vi "svx_Orbit Property Dialog.vi"(6 "Action in":T3 caption="Action", 7 "State in":T4={"X Scale"={"Name"="Horizontal", "FString"="%#.2g", "Major Color"=16777238, "Minor Color"=16777216, "Scale Visible"=TRUE, " Label Visible"=TRUE, "Grid Style"=1}, "Y Scale"={"Name"="Vertical", "FString"="%#.2g", "Major Color"=16777238, "Minor Color"=16777216, "Scale Visible"=TRUE, " Label Visible"=TRUE, "Grid Style"=1}, "Plot"={"Point Style"=0, "Line Width"=0, "Line Style"=0, "Plot Color"=9727, "Point/fill"=0}, "Arrow/Crosshair Color"=9727, "Tacho Point Color"=16711680, "Container Bounds"={"Width"=563, "Height"=294}, "Axis Maximum"=10.0, "Probe Angles"={"Angle X"=0.0, "Angle Y"=1.5707963267948966}, "Background Color"=16777226, "Cursor"={"Cursor Point Style"=13, "Cursor Style"=4, "Cursor Line Width"=1, "Cursor Line Style"=0, "Cursor Color"=9727, "Cursor Name Visible"=TRUE, "Cursor Visible"=TRUE, "Cursor Position"={"X"=0.0, "Y"=0.0}, "Cursor Index"=0, "Cursor Lock"=FALSE}, "Elliptical Info"=[], "Legend Visible"=TRUE, "Scale Range Change"=refnum, "Strings[]"={"Custom pair name"=FALSE, "Row Strings []"=[], "Column Strings []"=[]}, "Index"=[{"pair index"=0, "order index"=0}], " Parents Tags"=[], "Children Tags"=[], "Open?"=[], "Label"="", "Legend Width"=120, "Pair Strings Changed?"=FALSE, "Size"=[], "Legend Background"=16777226, "Legend Font"=16777222, "Cursor Release"=refnum, "Autoscale"=TRUE, "Precession Direction"=[], "Item Width"=0, "User Pair Strings []"=[], "Users Order Strings []"=[], "Autoscale Once"=TRUE, "Property Write"=refnum} caption="State" {"Index"."order index" min=0; "Index"."pair index" min=0; "Axis Maximum" min=0.0}, 8 "Ref In":T1, 11 "Orbit Plot":T2) -> (4 "Action out":T3 caption="Action", 5 "State out":T4={"X Scale"={"Name"="Horizontal", "FString"="%#.2g", "Major Color"=16777238, "Minor Color"=16777216, "Scale Visible"=TRUE, " Label Visible"=TRUE, "Grid Style"=1}, "Y Scale"={"Name"="Vertical", "FString"="%#.2g", "Major Color"=16777238, "Minor Color"=16777216, "Scale Visible"=TRUE, " Label Visible"=TRUE, "Grid Style"=1}, "Plot"={"Point Style"=0, "Line Width"=0, "Line Style"=0, "Plot Color"=9727, "Point/fill"=0}, "Arrow/Crosshair Color"=9727, "Tacho Point Color"=16711680, "Container Bounds"={"Width"=563, "Height"=294}, "Axis Maximum"=10.0, "Probe Angles"={"Angle X"=0.0, "Angle Y"=1.5707963267948966}, "Background Color"=16777226, "Cursor"={"Cursor Point Style"=13, "Cursor Style"=4, "Cursor Line Width"=1, "Cursor Line Style"=0, "Cursor Color"=9727, "Cursor Name Visible"=TRUE, "Cursor Visible"=TRUE, "Cursor Position"={"X"=0.0, "Y"=0.0}, "Cursor Index"=0, "Cursor Lock"=FALSE}, "Elliptical Info"=[], "Legend Visible"=TRUE, "Scale Range Change"=refnum, "Strings[]"={"Custom pair name"=FALSE, "Row Strings []"=[], "Column Strings []"=[]}, "Index"=[{"pair index"=0, "order index"=0}], " Parents Tags"=[], "Children Tags"=[], "Open?"=[], "Label"="", "Legend Width"=120, "Pair Strings Changed?"=FALSE, "Size"=[], "Legend Background"=16777226, "Legend Font"=16777222, "Cursor Release"=refnum, "Autoscale"=TRUE, "Precession Direction"=[], "Item Width"=0, "User Pair Strings []"=[], "Users Order Strings []"=[], "Autoscale Once"=TRUE, "Property Write"=refnum} caption="State" {"Index"."order index" min=0; "Index"."pair index" min=0; "Axis Maximum" min=0.0})   [LabVIEW 2017, in "SVX Orbit.xctl"]
uses:
  <vilib>/addons/_XControls/Orbit Plot/SVX Orbit.xctl
  <vilib>/addons/_XControls/Orbit Plot/subVIs/svx_Orbit Internal State.ctl
  <vilib>/addons/_XControls/Orbit Plot/subVIs/svx_Orbit Bounds.ctl
  <vilib>/_xctls/Action.ctl
  <vilib>/addons/_XControls/Orbit Plot/subVIs/svx_Orbit Data.ctl
  <vilib>/addons/_XControls/Orbit Plot/subVIs/svx_Orbit Core States.ctl
  <vilib>/_xctls/XControlSupport.lvlib
panel:
  in  "Help":bool
  in  "Cancel":bool
  in  "OK":bool
  in  "Main Tab":T6(tab)
  in  "Plot Legend Font.Color":u32(colorbox)=16777222 caption="Legend font"
  in  "Plot Legend Background.Color":u32(colorbox)=16777226 caption="Legend background"
  in  "Background.Color":u32(colorbox) caption="Background"
  in  "Arrow/Crosshair.Color":u32(colorbox)=6618880 caption="Arrow/Crosshair"
  in  "Label.Visible":bool=TRUE
  in  "Label.Text":string="Orbit Plot"
  in  "Caption.Visible":bool
  in  "Caption.Text":string="Orbit Plot"
  in  "Enable State":T7(radio)
  in  "Format Selection":u16(ring) caption="Format selection" items=["Horizontal (X-Axis)", "Vertical (Y-Axis)"]
  in  "Hide trailing zeros":bool=TRUE
  in  "Digits":u8=2
  in  "Precision Type":u16(ring) items=["Digits of precision", "Significant digits"]
  in  "Type":i32(listbox)=2
  in  "Point/Fill.Color":u32(colorbox)=16777226 caption="Point/Fill"
  in  "Plot.Point Style":T8={"OK Button 17"=TRUE, "OK Button"=FALSE, "OK Button 2"=FALSE, "OK Button 3"=FALSE, "OK Button 4"=FALSE, "OK Button 5"=FALSE, "OK Button 6"=FALSE, "OK Button 7"=FALSE, "OK Button 8"=FALSE, "OK Button 9"=FALSE, "OK Button 10"=FALSE, "OK Button 11"=FALSE, "OK Button 12"=FALSE, "OK Button 13"=FALSE, "OK Button 14"=FALSE, "OK Button 15"=FALSE, "OK Button 16"=FALSE} caption="Point Style"
  in  "Line.Color":u32(colorbox) caption="Line"
  in  "Plot.Line Style":T9={"OK Button"=TRUE, "OK Button 2"=FALSE, "OK Button 3"=FALSE, "OK Button 4"=FALSE, "OK Button 5"=FALSE} caption="Line Style"
  in  "Plot.Line Width":T10={"OK Button 2"=TRUE, "OK Button 3"=FALSE, "OK Button 4"=FALSE, "OK Button 5"=FALSE, "OK Button 6"=FALSE, "OK Button 7"=FALSE} caption="Line Width"
  in  "Trigger Point.Color":u32(colorbox)=16711680 caption="Trigger point"
  in  "YGrid Style":u16(ring) caption="Grid Style and Colors"
  in  "XGrid Style":u16(ring) caption="Grid Style and Colors"
  in  "Minor Grid.Color":u32(colorbox)=13056 caption="Minor grid"
  in  "Major Grid.Color":u32(colorbox)=26112 caption="Major grid"
  in  "Scale Label.Visible":bool caption="Show scale label"
  in  "Maximum":dbl=10.0 format="%#.6g"
  in  "Minimum":dbl format="%#.6g"
  in  "Scale Fit":bool caption="Autoscale"
  in  "Scale.Visible":bool=TRUE caption="Show scale"
  in  "Scale Name":string caption="Name"
  in  "Scale Selection":u16(ring) items=["Horizontal (X-Axis)", "Vertical (Y-Axis)"]
  in  "Cursor Info Position.Lock":bool=TRUE
  in  "Cursor.Line Width":T10 caption="Cursor Line Width"
  in  "Cursor.Point Style":T8 caption="Cursor Point Style"
  in  "Cursor.Line Style":T9 caption="Cursor Line Style"
  in  "Cursor Info.Visible":bool caption="Show name"
  in  "Cursor.Style":T11 caption="Cursor Style"
  in  "Cursor.Color":u32(colorbox) caption="Cursor color"
  in  "Cursor.Visible":bool=TRUE
  in  "Tip strip":string
  in  "Description":string
  # "Caption"
  # "Label"
  # "Enabled State"
  # "Color Scheme"
  # "Orbit Plot"
  # "Colors"
  # "Cursor"
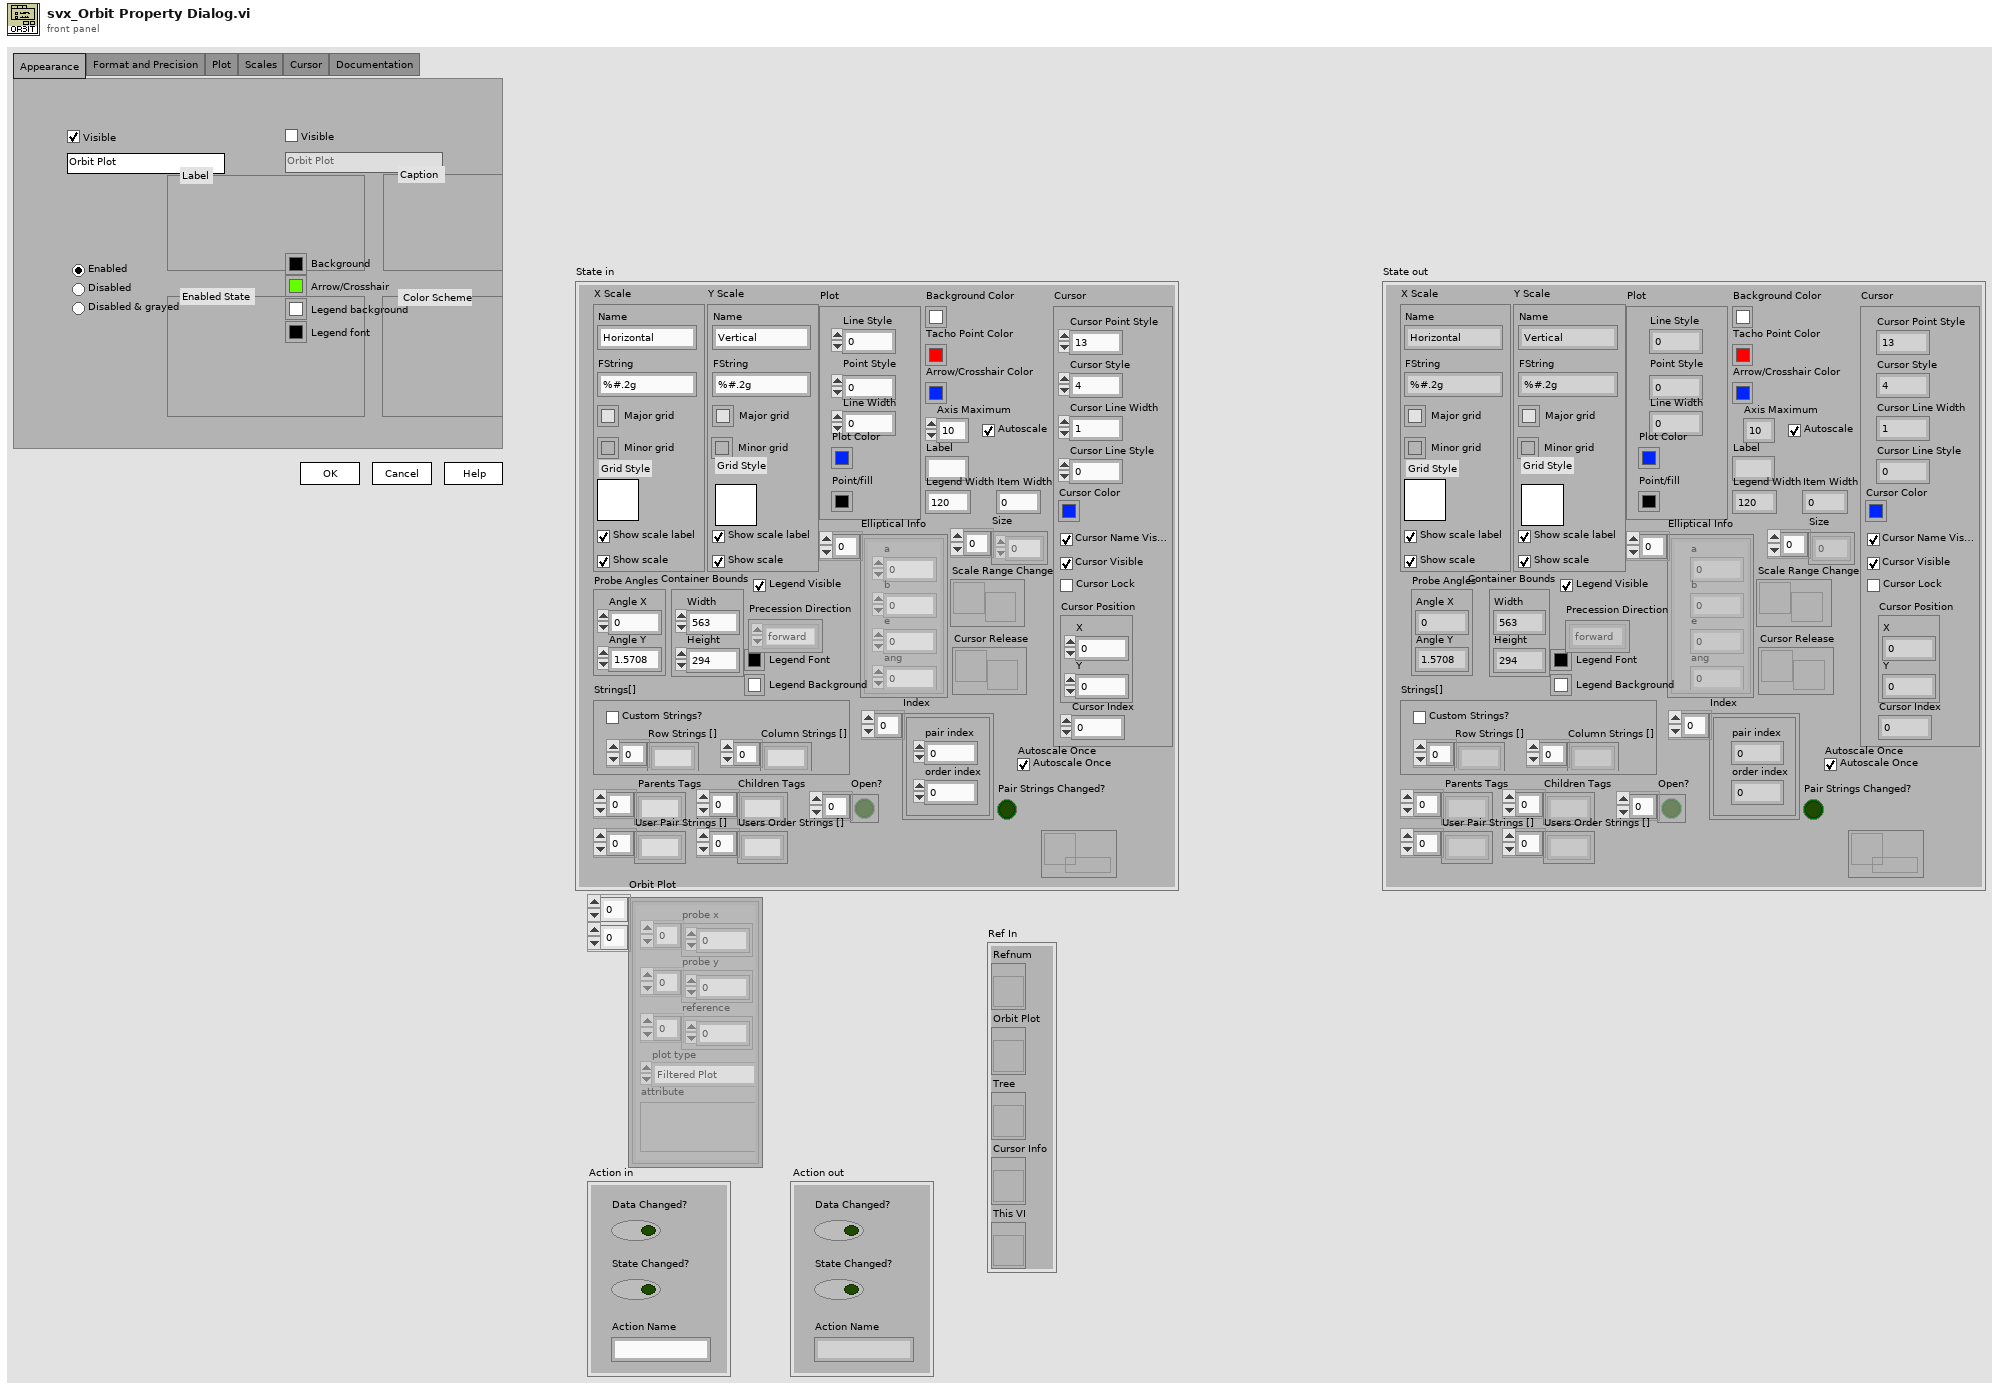
[diagram p1: front panel]
types:
  T1 = cluster{"Refnum":refnum<vi>, "Orbit Plot":refnum<vi>, "Tree":refnum<vi>, "Cursor Info":refnum<vi>, "This VI":refnum<vi>}
  T2 = typedef "SVX Orbit.xctl/svx_Orbit Data.ctl" = cluster{"probe x":dbl[], "probe y":dbl[], "reference":dbl[], "plot type":enum16{"Filtered Plot", "Unfiltered Plot"}, "attribute":variant}[][]
  T3 = typedef "XControlSupport.lvlib/Action.ctl" = cluster{"Data Changed?":bool, "State Changed?":bool, "Action Name":string}
  T4 = typedef "SVX Orbit.xctl/svx_Orbit Internal State.ctl" = cluster{"X Scale":cluster{"Name":string, "FString":string, "Major Color":u32, "Minor Color":u32, "Scale Visible":bool, " Label Visible":bool, "Grid Style":u16}, "Y Scale":cluster{"Name":string, "FString":string, "Major Color":u32, "Minor Color":u32, "Scale Visible":bool, " Label Visible":bool, "Grid Style":u16}, "Plot":cluster{"Point Style":u8, "Line Width":u8, "Line Style":u8, "Plot Color":u32, "Point/fill":u32}, "Arrow/Crosshair Color":u32, "Tacho Point Color":u32, "Container Bounds":T5, "Axis Maximum":dbl, "Probe Angles":cluster{"Angle X":dbl, "Angle Y":dbl}, "Background Color":u32, "Cursor":cluster{"Cursor Point Style":u8, "Cursor Style":u8, "Cursor Line Width":u8, "Cursor Line Style":u8, "Cursor Color":u32, "Cursor Name Visible":bool, "Cursor Visible":bool, "Cursor Position":cluster{"X":dbl, "Y":dbl}, "Cursor Index":i32, "Cursor Lock":bool}, "Elliptical Info":cluster{"a":dbl, "b":dbl, "e":dbl, "ang":dbl}[], "Legend Visible":bool, "Scale Range Change":refnum<user-event>, "Strings[]":cluster{"Custom pair name":bool, "Row Strings []":string[], "Column Strings []":string[]}, "Index":cluster{"pair index":i32, "order index":i32}[], " Parents Tags":string[], "Children Tags":string[], "Open?":bool[], "Label":string, "Legend Width":u32, "Pair Strings Changed?":bool, "Size":i32[], "Legend Background":u32, "Legend Font":u32, "Cursor Release":refnum<user-event>, "Autoscale":bool, "Precession Direction":enum16{"forward", "backward"}[], "Item Width":u32, "User Pair Strings []":string[], "Users Order Strings []":string[], "Autoscale Once":bool, "Property Write":refnum<queue>}
  T5 = typedef "SVX Orbit.xctl/svx_Orbit Bounds.ctl" = cluster{"Width":u32, "Height":u32}
  T6 = enum32{"Appearance", "Format and Precision", "Plot", "Scales", "Cursor", "Documentation"}
  T7 = enum32{"Enabled", "Disabled", "Disabled & grayed"}
  T8 = cluster{"OK Button 17":bool, "OK Button":bool, "OK Button 2":bool, "OK Button 3":bool, "OK Button 4":bool, "OK Button 5":bool, "OK Button 6":bool, "OK Button 7":bool, "OK Button 8":bool, "OK Button 9":bool, "OK Button 10":bool, "OK Button 11":bool, "OK Button 12":bool, "OK Button 13":bool, "OK Button 14":bool, "OK Button 15":bool, "OK Button 16":bool}
  T9 = cluster{"OK Button":bool, "OK Button 2":bool, "OK Button 3":bool, "OK Button 4":bool, "OK Button 5":bool}
  T10 = cluster{"OK Button 2":bool, "OK Button 3":bool, "OK Button 4":bool, "OK Button 5":bool, "OK Button 6":bool, "OK Button 7":bool}
  T11 = cluster{"OK Button 17":bool, "OK Button":bool, "OK Button 2":bool, "OK Button 5":bool, "OK Button 13":bool, "OK Button 10":bool, "OK Button 6":bool, "OK Button 9":bool, "OK Button 14":bool}
  T12 = cluster{"Desc":string, "TipStrip":string, "Label.Text":string, "Label.Visible":bool, "Caption.Text":string, "Caption.Visible":bool, "Disabled":u8}
  T13 = cluster{"probe x":dbl[], "probe y":dbl[], "reference":dbl[], "plot type":enum16{"Filtered Plot", "Unfiltered Plot"}, "attribute":variant}
  T14 = typedef "SVX Orbit.xctl/svx_Orbit Core States.ctl" = enum16{"None", "[Axis] Range", "[Plot] Image", "[Plot] Tacho Point", "[Plot] Grid and BG", "[Cursor] Cursor Info", "[Legend] Pair Strings", "[Data] Plot Data", "[Legend] Checkbox", "[Layout] Update", "[Legend] Tree Open", "[Layout] Legend Visible", "[Plot] Data Point", "[Axis] Axis and Label", "[Axis] Format String", "[Cursor] Appearance", "[Cursor] Index", "[Legend] Color", "[Layout] Min Pane Size", "[Data] Legend Strings"}
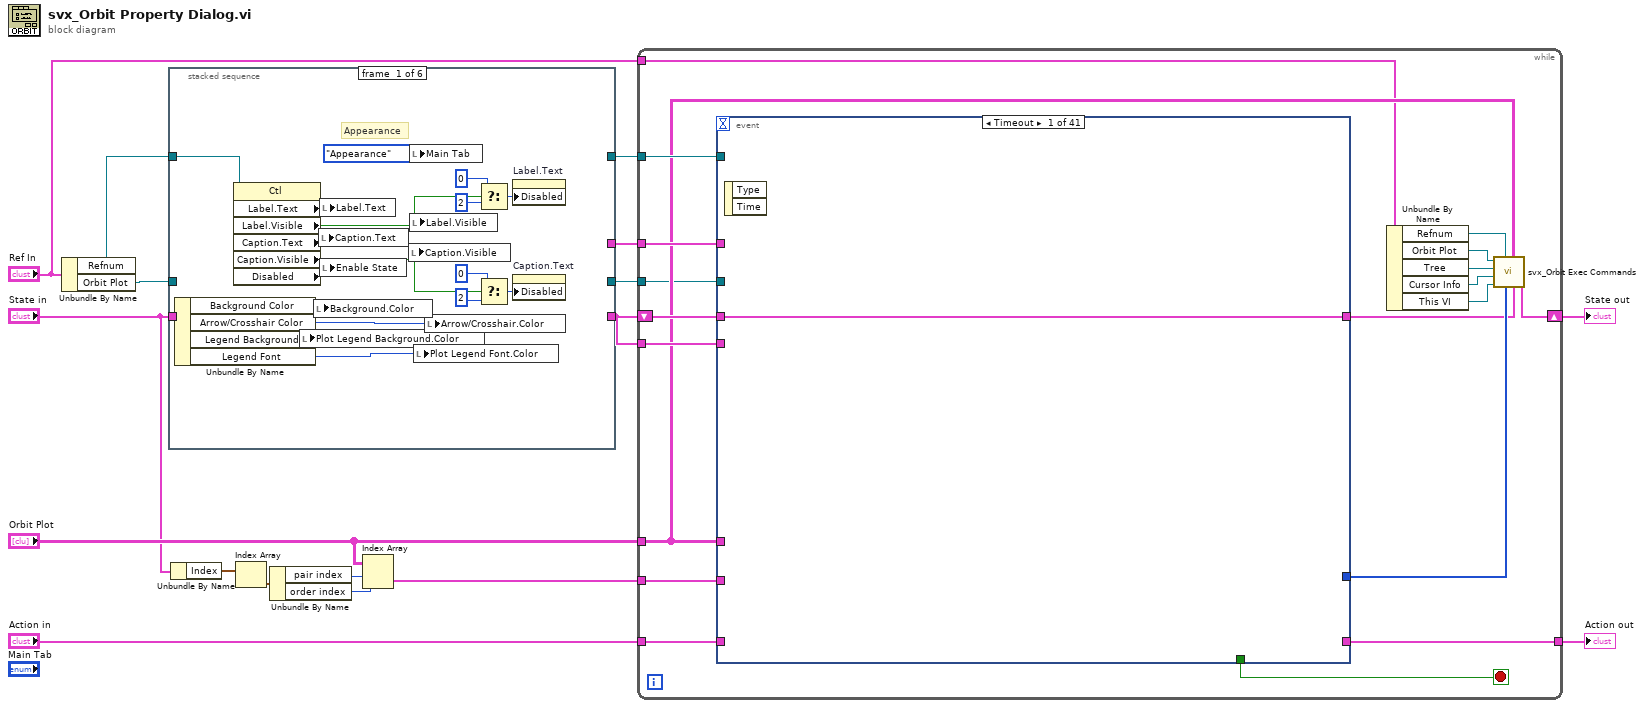
[diagram p0: block diagram]
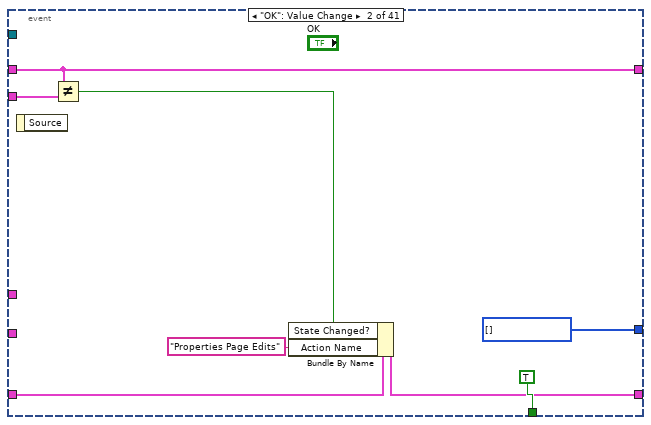
[diagram p2: hidden frame]
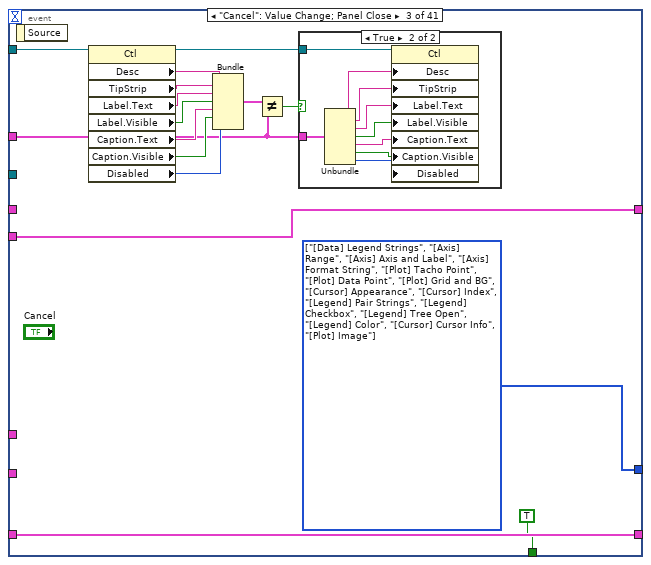
[diagram p3: hidden frame]
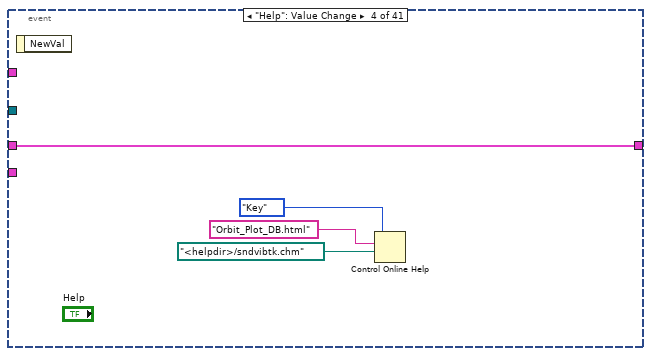
[diagram p5: hidden frame]
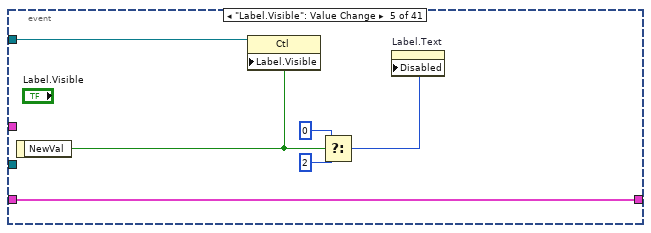
[diagram p6: hidden frame]
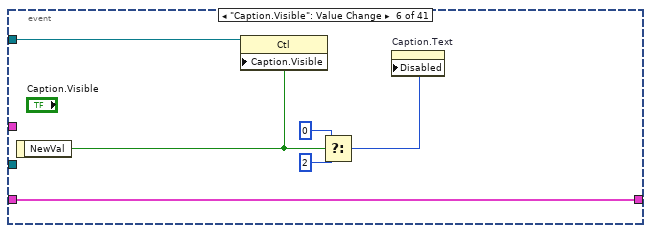
[diagram p7: hidden frame]
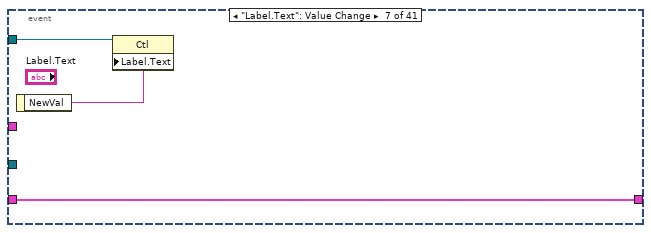
[diagram p8: hidden frame]
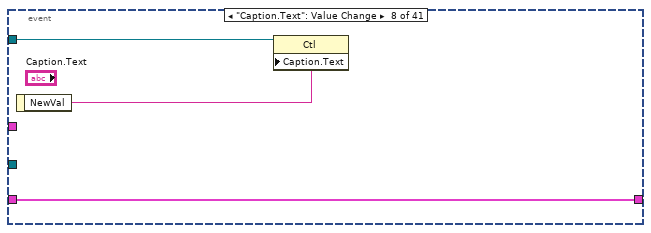
[diagram p9: hidden frame]
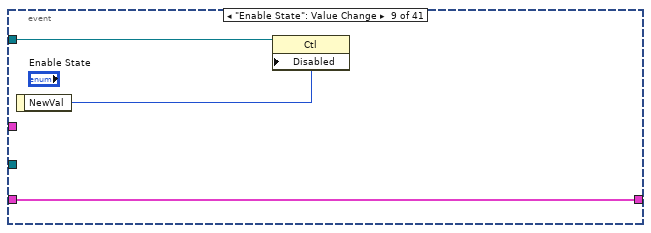
[diagram p10: hidden frame]
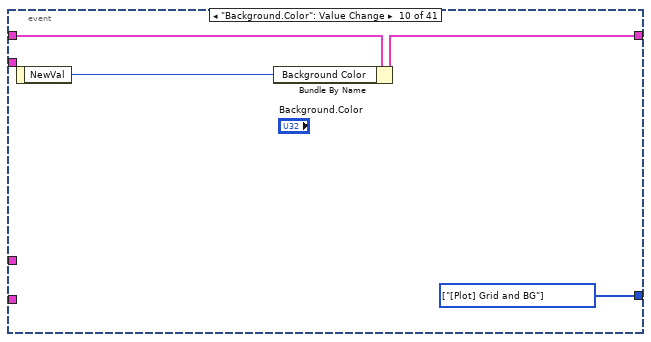
[diagram p11: hidden frame]
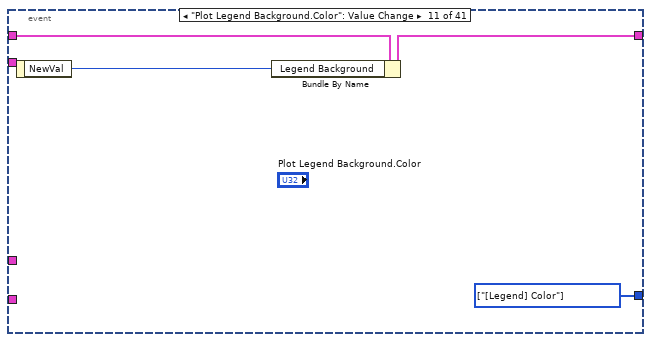
[diagram p12: hidden frame]
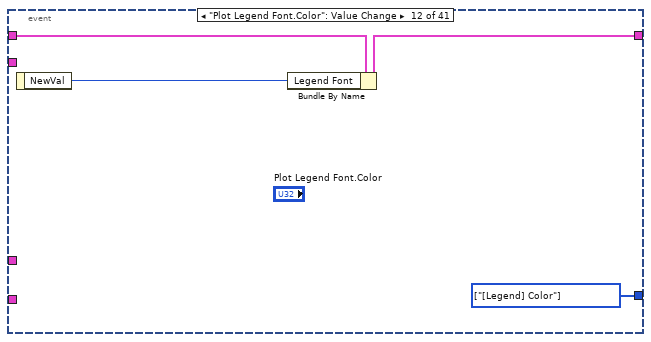
[diagram p13: hidden frame]
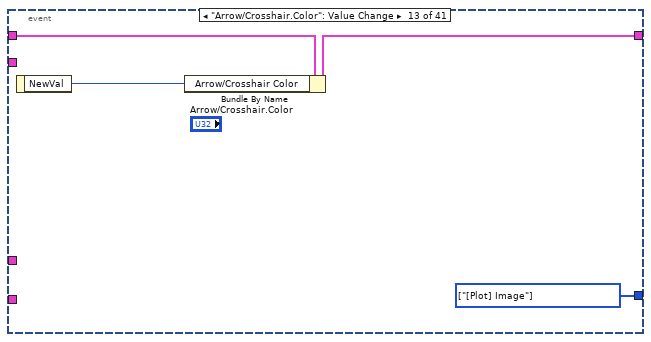
[diagram p14: hidden frame]
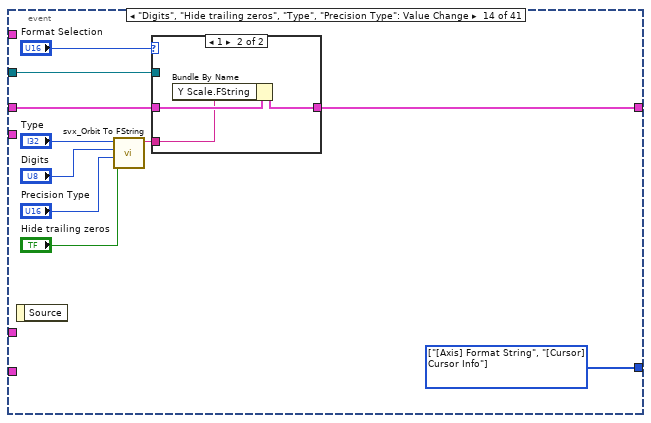
[diagram p15: hidden frame]
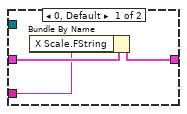
[diagram p16: hidden frame]
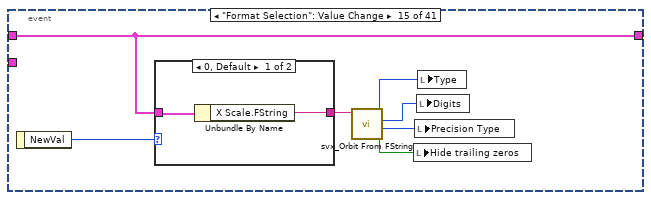
[diagram p17: hidden frame]
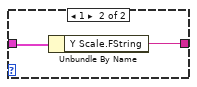
[diagram p18: hidden frame]
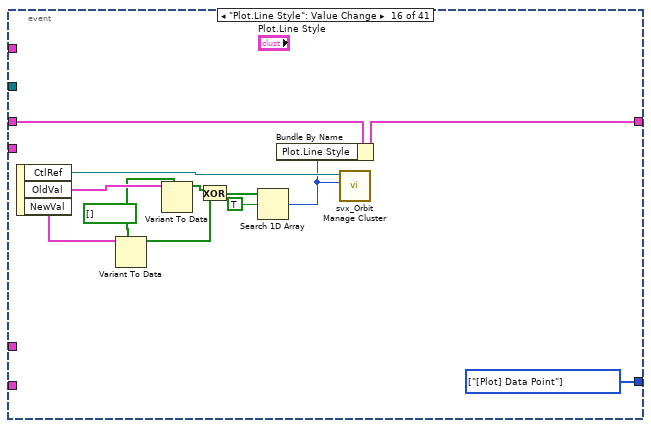
[diagram p19: hidden frame]
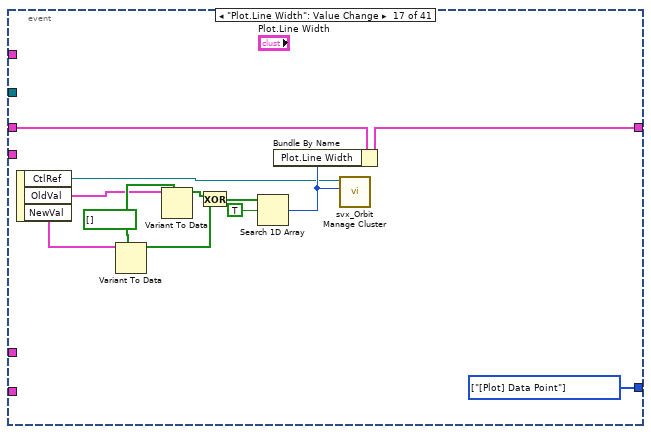
[diagram p20: hidden frame]
diagram:
  n1 = Unbundle By Name("Ref In") -> ("Refnum"=w3:refnum<vi>, "Orbit Plot"=w2:refnum<vi>)
  n2 = stacked-sequence {
    tunnel: w3 -> [w35 _ _ _ _ w118]
    tunnel: "State in" -> [w32 w41 w55 w78 w107 w119]
    tunnel: [_ _ _ _ _ w117] -> w17
    tunnel: [_ _ _ _ _ w119] -> w16
    tunnel: [_ _ _ _ _ w108] -> w14
    tunnel: w2 -> [_ _ _ _ _ w108]
    tunnel: [_ _ _ _ _ w109] -> w13
    frame #0 {
      # "Appearance"
      n3 = Unbundle By Name(w32) -> ("Background Color"=w34:u32, "Arrow/Crosshair Color"=w33:u32, "Legend Background"=w19:u32, "Legend Font"=w18:u32)
      n4 = property class="Ctl"(reference=w35) -> ("Label.Text"=w26:string, "Label.Visible"=w25:bool, "Caption.Text"=w24:string, "Caption.Visible"=w22:bool, "Disabled"=w23:u8)  [unwired: 1 in, 2 out]
      n5 = local write "Plot Legend Background.Color"(w19) -> ()
      n6 = local write "Background.Color"(w34) -> ()
      n7 = local write "Caption.Text"(w24) -> ()
      n8 = local write "Label.Text"(w26) -> ()
      n9 = local write "Enable State"(w23) -> ()
      n10 = local write "Caption.Visible"(w22) -> ()
      n11 = local write "Main Tab"(T6."Appearance" ("Main Tab")) -> ()
      n12 = local write "Label.Visible"(w25) -> ()
      n13 = local write "Plot Legend Font.Color"(w18) -> ()
      n14 = local write "Arrow/Crosshair.Color"(w33) -> ()
      n15 = Select(t=u8 0 ("Disabled"), s=w25, f=u8 2) -> (s? t:f=w30:u8)
      n16 = Select(t=u8 0 ("Disabled"), s=w22, f=u8 2) -> (s? t:f=w27:u8)
      n17 = property on="Label.Text" class="Str"("Disabled"=w30) -> ()  [unwired: 2 in, 2 out]
      n18 = property on="Caption.Text" class="Str"("Disabled"=w27) -> ()  [unwired: 2 in, 2 out]
    }
    frame #1 {
      w42 = u16 0 items=["X-Axis", "Y-Axis"] ("Format selection")
      # "Format and Precision"
      n19 = Unbundle By Name(w41) -> ("X Scale.FString"=w40:string)
      n20 = call <vilib>:"svx_Orbit From FString.vi"("Format string"=w40) -> ("trailing zeros"=w36:bool, "Precision Type"=w37:u16, "Digits"=w38:u8, "Type"=w39:i32)  [unwired: 7 in]
      n21 = local write "Format Selection"(w42) -> ()
      n22 = local write "Hide trailing zeros"(w36) -> ()
      n23 = local write "Precision Type"(w37) -> ()
      n24 = local write "Digits"(w38) -> ()
      n25 = local write "Type"(w39) -> ()
    }
    frame #2 {
      # "Plot"
      n26 = Unbundle By Name(w55) -> ("Plot.Plot Color"=w48:u32, "Tacho Point Color"=w47:u32, "Plot.Point/fill"=w46:u32, "Plot.Line Width"=w54:u8, "Plot.Line Style"=w52:u8, "Plot.Point Style"=w51:u8)
      n27 = control-ref of="Plot.Line Width"() -> (w53:refnum<vi>)
      n28 = control-ref of="Plot.Line Style"() -> (w49:refnum<vi>)
      n29 = control-ref of="Plot.Point Style"() -> (w50:refnum<vi>)
      n30 = To Long Integer(number=w54) -> (32bit integer=w43:i32)
      n31 = To Long Integer(number=w52) -> (32bit integer=w44:i32)
      n32 = To Long Integer(number=w51) -> (32bit integer=w45:i32)
      n33 = local write "Point/Fill.Color"(w46) -> ()
      n34 = local write "Trigger Point.Color"(w47) -> ()
      n35 = call <vilib>:"svx_Orbit Manage Cluster.vi"("index"=w43, "Clust Refnum"=w53) -> ()  [unwired: 10 in]
      n36 = call <vilib>:"svx_Orbit Manage Cluster.vi"("index"=w44, "Clust Refnum"=w49) -> ()  [unwired: 10 in]
      n37 = call <vilib>:"svx_Orbit Manage Cluster.vi"("index"=w45, "Clust Refnum"=w50) -> ()  [unwired: 10 in]
      n38 = local write "Line.Color"(w48) -> ()
    }
    frame #3 {
      w79 = u16 0 items=["X-Axis", "Y-Axis"] ("Scale selection")
      # "Scales"
      n39 = Unbundle By Name(w78) -> ("Y Scale.Name"=w60:string, "X Scale.Name"=w58:string, "X Scale.Label Visible"=w77:bool, "X Scale.Scale Visible"=w76:bool, "X Scale.Grid Style"=w66:u16, "X Scale.Major Color"=w75:u32, "X Scale.Minor Color"=w74:u32, "Autoscale"=w56:bool, "Axis Maximum"=w62:dbl)
      n40 = local write "Scale Selection"(w79) -> ()
      n41 = property on="YGrid Style" class="Ring (strict)"("Visible"=FALSE) -> ()  [unwired: 2 in, 2 out]
      n42 = property on="XGrid Style" class="Ring (strict)"("Visible"=TRUE) -> ()  [unwired: 2 in, 2 out]
      n43 = Concatenate Strings(w60, " (Y-Axis)" ("string")) -> (w63:string)
      n44 = Negate(x=w62) -> (-x=w73:dbl)
      n45 = local write "Minimum"(w73) -> ()
      n46 = local write "Scale Label.Visible"(w77) -> ()
      n47 = local write "Maximum"(w62) -> ()
      n48 = local write "Minor Grid.Color"(w74) -> ()
      n49 = local write "XGrid Style"(w66) -> ()
      n50 = case shown="1" w66 {
        tunnel: [w80 u8 0 ("Disabled") w83] -> w68
        tunnel: [w80 u8 2 ("Disabled") w83] -> w67
        frame 0, Default {
          w80 = u8 2 ("Disabled")
        }
        frame 1 {
        }
        frame 2 {
          w83 = u8 0 ("Disabled")
        }
      }
      n51 = Concatenate Strings(w58, " (X-Axis)" ("string")) -> (w64:string)
      n52 = Build Array(w64, w63) -> (w61:string[])
      n53 = Select(t=u8 2 ("Disabled"), s=w56, f=u8 0) -> (s? t:f=w70:u8)
      n54 = local write "Scale Name"(w58) -> ()
      n55 = local write "Scale.Visible"(w76) -> ()
      n56 = local write "Major Grid.Color"(w75) -> ()
      n57 = local write "Scale Fit"(w56) -> ()
      n58 = property on="Minimum" class="DigNum (strict)"("Disabled"=w70) -> ()  [unwired: 2 in, 2 out]
      n59 = property on="Maximum" class="DigNum (strict)"("Disabled"=w70) -> ()  [unwired: 2 in, 2 out]
      n60 = property on="Major Grid.Color" class="ColBox"("Disabled"=w68) -> ()  [unwired: 2 in, 2 out]
      n61 = property on="Minor Grid.Color" class="ColBox"("Disabled"=w67) -> ()  [unwired: 2 in, 2 out]
      n62 = property on="Format Selection" class="Ring (strict)"("Strings []"=w61) -> ()  [unwired: 2 in, 2 out]
      n63 = property on="Scale Selection" class="Ring (strict)"("Strings []"=w61) -> ()  [unwired: 2 in, 2 out]
    }
    frame #4 {
      # "Cursor"
      n64 = Unbundle By Name(w107) -> ("Cursor.Cursor Point Style"=w106:u8, "Cursor.Cursor Style"=w104:u8, "Cursor.Cursor Line Width"=w102:u8, "Cursor.Cursor Line Style"=w100:u8, "Cursor.Cursor Color"=w98:u32, "Cursor.Cursor Name Visible"=w90:bool, "Cursor.Cursor Visible"=w89:bool, "Cursor.Cursor Lock"=w97:bool)
      n65 = And(x=w90, y=w89) -> (x .and. y?=w88:bool)
      n66 = local write "Cursor Info Position.Lock"(w97) -> ()
      n67 = local write "Cursor Info.Visible"(w90) -> ()
      n68 = To Long Integer(number=w104) -> (32bit integer=w85:i32)
      n69 = To Long Integer(number=w100) -> (32bit integer=w87:i32)
      n70 = control-ref of="Cursor.Point Style"() -> (w105:refnum<vi>)
      n71 = control-ref of="Cursor.Style"() -> (w103:refnum<vi>)
      n72 = control-ref of="Cursor.Line Style"() -> (w99:refnum<vi>)
      n73 = Select(t=u8 0 ("Disabled"), s=w89, f=u8 2) -> (s? t:f=w94:u8)
      n74 = Select(t=u8 0 ("Disabled"), s=w88, f=u8 2) -> (s? t:f=w93:u8)
      n75 = call <vilib>:"svx_Orbit Manage Cluster.vi"("index"=w85, "Clust Refnum"=w103) -> ()  [unwired: 10 in]
      n76 = call <vilib>:"svx_Orbit Manage Cluster.vi"("index"=w87, "Clust Refnum"=w99) -> ()  [unwired: 10 in]
      n77 = To Long Integer(number=w106) -> (32bit integer=w84:i32)
      n78 = To Long Integer(number=w102) -> (32bit integer=w86:i32)
      n79 = control-ref of="Cursor.Line Width"() -> (w101:refnum<vi>)
      n80 = local write "Cursor.Visible"(w89) -> ()
      n81 = local write "Cursor.Color"(w98) -> ()
      n82 = property on="Cursor Info.Visible" class="Bool (strict)"("Disabled"=w94) -> ()  [unwired: 2 in, 2 out]
      n83 = property on="Cursor Info Position.Lock" class="Bool (strict)"("Disabled"=w93) -> ()  [unwired: 2 in, 2 out]
      n84 = call <vilib>:"svx_Orbit Manage Cluster.vi"("index"=w84, "Clust Refnum"=w105) -> ()  [unwired: 10 in]
      n85 = call <vilib>:"svx_Orbit Manage Cluster.vi"("index"=w86, "Clust Refnum"=w101) -> ()  [unwired: 10 in]
    }
    frame #5 {
      n86 = property class="Ctl"(reference=w118) -> (reference out=w117:refnum<vi>, "Desc"=w110:string, "TipStrip"=w111:string, "Label.Text"=w116:string, "Label.Visible"=w115:bool, "Caption.Text"=w114:string, "Caption.Visible"=w113:bool, "Disabled"=w112:u8)  [unwired: 1 in, 1 out]
      n87 = local write "Description"(w110) -> ()
      n88 = local write "Tip strip"(w111) -> ()
      n89 = Bundle("Desc"=w110, "TipStrip"=w111, "Label.Text"=w116, "Label.Visible"=w115, "Caption.Text"=w114, "Caption.Visible"=w113, "Disabled"=w112) -> (w109:T12)  [unwired: 1 in]
    }
  }
  n90 = Unbundle By Name("State in") -> ("Index"=w8:cluster{"pair index":i32, "order index":i32}[])
  n91 = Index Array(array=w8) -> (element=w7:cluster{"pair index":i32, "order index":i32})  [unwired: 1 in]
  n92 = Unbundle By Name(w7) -> ("pair index"=w6:i32, "order index"=w5:i32)
  n93 = Index Array(array="Orbit Plot", index (row)=w6, index (col)=w5) -> (element=w9:T13)
  n94 = while {
    tunnel: w17 -> [w135]
    shift-right: [w129] -> w12
    shift-left: w16 -> [w137]
    tunnel: w16 -> [w133]
    tunnel: w14 -> [w126]
    tunnel: w13 -> [w134]
    tunnel: "Orbit Plot" -> [w128]
    tunnel: w9 -> [w132]
    tunnel: "Action in" -> [w136]
    tunnel: [w127] -> w4
    tunnel: "Ref In" -> [w125]
    stop <- w138 stop-if-true
    n95 = event shown="[0] Timeout" {
      selector: _ -> [_ _ _ _ _ _ _ _ _ _ _ _ _ _ _ _ _ _ _ _ _ _ _ _ _ _ _ _ _ _ _ _ _ _ _ _ _ _ _ _ _]
      dyn-events: _ -> [_ _ _ _ _ _ _ _ _ _ _ _ _ _ _ _ _ _ _ _ _ _ _ _ _ _ _ _ _ _ _ _ _ _ _ _ _ _ _ _ _]
      timeout: _ -> [_ _ _ _ _ _ _ _ _ _ _ _ _ _ _ _ _ _ _ _ _ _ _ _ _ _ _ _ _ _ _ _ _ _ _ _ _ _ _ _ _]
      tunnel: [_ TRUE TRUE _ _ _ _ _ _ _ _ _ _ _ _ _ _ _ _ _ _ _ _ _ _ _ _ _ _ _ _ _ _ _ _ _ _ _ _ _ _] -> w138
      tunnel: w137 -> [w139 w140 _ w173 w177 w183 w189 w192 w195 w201 w205 w209 w212 w216 w235 w244 w259 w271 w280 w284 w288 w297 w310 w321 w331 w343 w349 w359 w369 w380 w389 w435 w447 w459 w471 w483 w485 w499 w503 w504 w507]
      tunnel: w133 -> [_ w146 w161 _ _ _ _ _ _ _ _ _ _ _ _ _ _ _ _ _ _ _ _ _ _ _ _ _ _ _ _ _ _ _ _ _ _ _ _ _ _]
      tunnel: w136 -> [_ w145 w163 _ _ _ _ _ _ _ _ _ _ _ _ _ _ _ _ _ _ _ _ _ _ _ _ _ _ _ _ _ _ _ _ _ _ _ _ _ _]
      tunnel: [_ w144 w163 _ _ _ _ _ _ _ _ _ _ _ _ _ _ _ _ _ _ _ _ _ _ _ _ _ _ _ _ _ _ _ _ _ _ _ _ _ _] -> w127
      tunnel: [_ w141 w160 _ _ _ _ _ _ w198 w202 w206 w210 w214 _ w241 w253 w265 w277 w281 w285 w289 w306 w317 _ w338 w348 w355 w365 w376 _ w429 w441 w453 w465 w477 w486 w496 w500 _ _] -> w131
      tunnel: w126 -> [_ _ _ _ _ _ _ _ _ _ _ _ _ w218 _ _ _ _ _ _ _ _ _ _ w337 _ _ _ _ _ _ _ _ _ _ _ _ _ _ _ _]
      tunnel: w135 -> [_ _ w148 _ w182 w188 w191 w194 w197 _ _ _ _ _ _ _ _ _ _ _ _ _ _ _ _ _ _ _ _ _ _ _ _ _ _ _ _ _ _ w506 w509]
      tunnel: w134 -> [_ _ w149 _ _ _ _ _ _ _ _ _ _ _ _ _ _ _ _ _ _ _ _ _ _ _ _ _ _ _ _ _ _ _ _ _ _ _ _ _ _]
      tunnel: [w139 w140 w161 w173 w177 w183 w189 w192 w195 w200 w203 w208 w213 w215 w235 w243 w258 w270 w279 w283 w287 w296 w309 w320 w329 w340 w350 w360 w368 w379 w389 w434 w446 w458 w470 w482 w495 w498 w501 w504 w507] -> w130
      tunnel: w128 -> [_ _ _ _ _ _ _ _ _ _ _ _ _ _ _ _ _ _ _ _ _ _ _ _ _ _ _ _ _ _ _ _ _ _ _ _ _ _ _ _ _]
      tunnel: w132 -> [_ _ _ _ _ _ _ _ _ _ _ _ _ _ _ _ _ _ _ _ _ _ _ _ w333 _ _ _ _ _ _ _ _ _ _ _ _ _ _ _ _]
      event Timeout {
        n96 = event-data() -> ()  [unwired: 1 in, 2 out]
      }
      event "OK": Value Change {
        w141 = T14[] [] items=["None", "[Axis] Range", "[Plot] Image", "[Plot] Tacho Point", "[Plot] Grid and BG", "[Cursor] Cursor Info", "[Legend] Pair Strings", "[Data] Plot Data", "[Legend] Checkbox", "[Layout] Update", "[Legend] Tree Open", "[Layout] Legend Visible", "[Plot] Data Point", "[Axis] Axis and Label", "[Axis] Format String", "[Cursor] Appearance", "[Cursor] Index", "[Legend] Color", "[Layout] Min Pane Size", "[Data] Legend Strings"] ("event")
        n97 = event-data() -> ()  [unwired: 1 in, 1 out]
        n98 = Not Equal?(x=w140, y=w146) -> (x != y?=w143:bool)
        n99 = Bundle By Name(cluster=w145, "State Changed?"=w143, "Action Name"="Properties Page Edits") -> (w144:T3)
      }
      event "Cancel": Value Change; Panel Close {
        w160 = T14[] [enum."[Data] Legend Strings", enum."[Axis] Range", enum."[Axis] Axis and Label", enum."[Axis] Format String", enum."[Plot] Tacho Point", enum."[Plot] Data Point", enum."[Plot] Grid and BG", enum."[Cursor] Appearance", enum."[Cursor] Index", enum."[Legend] Pair Strings", enum."[Legend] Checkbox", enum."[Legend] Tree Open", enum."[Legend] Color", enum."[Cursor] Cursor Info", enum."[Plot] Image"] items=["None", "[Axis] Range", "[Plot] Image", "[Plot] Tacho Point", "[Plot] Grid and BG", "[Cursor] Cursor Info", "[Legend] Pair Strings", "[Data] Plot Data", "[Legend] Checkbox", "[Layout] Update", "[Legend] Tree Open", "[Layout] Legend Visible", "[Plot] Data Point", "[Axis] Axis and Label", "[Axis] Format String", "[Cursor] Appearance", "[Cursor] Index", "[Legend] Color", "[Layout] Min Pane Size", "[Data] Legend Strings"]
        n100 = event-data() -> ()  [unwired: 1 in, 1 out]
        n101 = property class="Ctl"(reference=w148) -> (reference out=w159:refnum<vi>, "Desc"=w158:string, "TipStrip"=w157:string, "Label.Text"=w156:string, "Label.Visible"=w155:bool, "Caption.Text"=w154:string, "Caption.Visible"=w153:bool, "Disabled"=w152:u8)  [unwired: 1 in, 1 out]
        n102 = Bundle("Desc"=w158, "TipStrip"=w157, "Label.Text"=w156, "Label.Visible"=w155, "Caption.Text"=w154, "Caption.Visible"=w153, "Disabled"=w152) -> (w151:T12)  [unwired: 1 in]
        n103 = Not Equal?(x=w151, y=w149) -> (x != y?=w150:bool)
        n104 = case shown="True" w150 {
          tunnel: w159 -> [_ w165]
          tunnel: w149 -> [_ w164]
          frame False {
          }
          frame True {
            n105 = Unbundle(w164) -> ("Desc"=w172:string, "TipStrip"=w171:string, "Label.Text"=w170:string, "Label.Visible"=w169:bool, "Caption.Text"=w168:string, "Caption.Visible"=w167:bool, "Disabled"=w166:u8)
            n106 = property class="Ctl"(reference=w165, "Desc"=w172, "TipStrip"=w171, "Label.Text"=w170, "Label.Visible"=w169, "Caption.Text"=w168, "Caption.Visible"=w167, "Disabled"=w166) -> ()  [unwired: 1 in, 2 out]
          }
        }
      }
      event "Help": Value Change {
        n107 = event-data() -> ()  [unwired: 1 in, 1 out]
        n108 = Control Online Help(2:path "<helpdir>/sndvibtk.chm" ("Path to the help file"), 3:"Orbit_Plot_DB.html" ("String to search for"), 4:enum16{"Contents", "Key", "Close"}."Key" ("Operation")) -> ()  [unwired: 1 in, 1 out]
      }
      event "Label.Visible": Value Change {
        n109 = event-data() -> ("NewVal"=w179:bool)  [unwired: 1 in]
        n110 = property class="Ctl"(reference=w182, "Label.Visible"=w179) -> ()  [unwired: 1 in, 2 out]
        n111 = Select(t=u8 0 ("Disabled"), s=w179, f=u8 2) -> (s? t:f=w178:u8)
        n112 = property on="Label.Text" class="Str"("Disabled"=w178) -> ()  [unwired: 2 in, 2 out]
      }
      event "Caption.Visible": Value Change {
        n113 = event-data() -> ("NewVal"=w185:bool)  [unwired: 1 in]
        n114 = property class="Ctl"(reference=w188, "Caption.Visible"=w185) -> ()  [unwired: 1 in, 2 out]
        n115 = Select(t=u8 0 ("Disabled"), s=w185, f=u8 2) -> (s? t:f=w184:u8)
        n116 = property on="Caption.Text" class="Str"("Disabled"=w184) -> ()  [unwired: 2 in, 2 out]
      }
      event "Label.Text": Value Change {
        n117 = event-data() -> ("NewVal"=w190:string)  [unwired: 1 in]
        n118 = property class="Ctl"(reference=w191, "Label.Text"=w190) -> ()  [unwired: 1 in, 2 out]
      }
      event "Caption.Text": Value Change {
        n119 = event-data() -> ("NewVal"=w193:string)  [unwired: 1 in]
        n120 = property class="Ctl"(reference=w194, "Caption.Text"=w193) -> ()  [unwired: 1 in, 2 out]
      }
      event "Enable State": Value Change {
        n121 = event-data() -> ("NewVal"=w196:T7)  [unwired: 1 in]
        n122 = property class="Ctl"(reference=w197, "Disabled"=w196) -> ()  [unwired: 1 in, 2 out]
      }
      event "Background.Color": Value Change {
        w198 = T14[] [enum."[Plot] Grid and BG"] items=["None", "[Axis] Range", "[Plot] Image", "[Plot] Tacho Point", "[Plot] Grid and BG", "[Cursor] Cursor Info", "[Legend] Pair Strings", "[Data] Plot Data", "[Legend] Checkbox", "[Layout] Update", "[Legend] Tree Open", "[Layout] Legend Visible", "[Plot] Data Point", "[Axis] Axis and Label", "[Axis] Format String", "[Cursor] Appearance", "[Cursor] Index", "[Legend] Color", "[Layout] Min Pane Size", "[Data] Legend Strings"] ("event")
        n123 = event-data() -> ("NewVal"=w199:u32)  [unwired: 1 in]
        n124 = Bundle By Name(cluster=w201, "Background Color"=w199) -> (w200:T4)
      }
      event "Plot Legend Background.Color": Value Change {
        w202 = T14[] [enum."[Legend] Color"] items=["None", "[Axis] Range", "[Plot] Image", "[Plot] Tacho Point", "[Plot] Grid and BG", "[Cursor] Cursor Info", "[Legend] Pair Strings", "[Data] Plot Data", "[Legend] Checkbox", "[Layout] Update", "[Legend] Tree Open", "[Layout] Legend Visible", "[Plot] Data Point", "[Axis] Axis and Label", "[Axis] Format String", "[Cursor] Appearance", "[Cursor] Index", "[Legend] Color", "[Layout] Min Pane Size", "[Data] Legend Strings"] ("event")
        n125 = event-data() -> ("NewVal"=w204:u32)  [unwired: 1 in]
        n126 = Bundle By Name(cluster=w205, "Legend Background"=w204) -> (w203:T4)
      }
      event "Plot Legend Font.Color": Value Change {
        w206 = T14[] [enum."[Legend] Color"] items=["None", "[Axis] Range", "[Plot] Image", "[Plot] Tacho Point", "[Plot] Grid and BG", "[Cursor] Cursor Info", "[Legend] Pair Strings", "[Data] Plot Data", "[Legend] Checkbox", "[Layout] Update", "[Legend] Tree Open", "[Layout] Legend Visible", "[Plot] Data Point", "[Axis] Axis and Label", "[Axis] Format String", "[Cursor] Appearance", "[Cursor] Index", "[Legend] Color", "[Layout] Min Pane Size", "[Data] Legend Strings"] ("event")
        n127 = event-data() -> ("NewVal"=w207:u32)  [unwired: 1 in]
        n128 = Bundle By Name(cluster=w209, "Legend Font"=w207) -> (w208:T4)
      }
      event "Arrow/Crosshair.Color": Value Change {
        w210 = T14[] [enum."[Plot] Image"] items=["None", "[Axis] Range", "[Plot] Image", "[Plot] Tacho Point", "[Plot] Grid and BG", "[Cursor] Cursor Info", "[Legend] Pair Strings", "[Data] Plot Data", "[Legend] Checkbox", "[Layout] Update", "[Legend] Tree Open", "[Layout] Legend Visible", "[Plot] Data Point", "[Axis] Axis and Label", "[Axis] Format String", "[Cursor] Appearance", "[Cursor] Index", "[Legend] Color", "[Layout] Min Pane Size", "[Data] Legend Strings"] ("event")
        n129 = event-data() -> ("NewVal"=w211:u32)  [unwired: 1 in]
        n130 = Bundle By Name(cluster=w212, "Arrow/Crosshair Color"=w211) -> (w213:T4)
      }
      event "Digits", "Hide trailing zeros", "Type", "Precision Type": Value Change {
        w214 = T14[] [enum."[Axis] Format String", enum."[Cursor] Cursor Info"] items=["None", "[Axis] Range", "[Plot] Image", "[Plot] Tacho Point", "[Plot] Grid and BG", "[Cursor] Cursor Info", "[Legend] Pair Strings", "[Data] Plot Data", "[Legend] Checkbox", "[Layout] Update", "[Legend] Tree Open", "[Layout] Legend Visible", "[Plot] Data Point", "[Axis] Axis and Label", "[Axis] Format String", "[Cursor] Appearance", "[Cursor] Index", "[Legend] Color", "[Layout] Min Pane Size", "[Data] Legend Strings"] ("event")
        n131 = event-data() -> ()  [unwired: 1 in, 1 out]
        n132 = call <vilib>:"svx_Orbit To FString.vi"("trailing zeros"="Hide trailing zeros", "Precision Type"="Precision Type", "Digits"="Digits", "Type"="Type") -> ("format string"=w217:string)  [unwired: 7 in]
        n133 = case shown="1" "Format Selection" {
          tunnel: w218 -> [_ _]
          tunnel: w217 -> [w224 w227]
          tunnel: w216 -> [w226 w229]
          tunnel: [w225 w228] -> w215
          frame 0, Default {
            n134 = Bundle By Name(cluster=w226, "X Scale.FString"=w224) -> (w225:T4)
          }
          frame 1 {
            n135 = Bundle By Name(cluster=w229, "Y Scale.FString"=w227) -> (w228:T4)
          }
        }
      }
      event "Format Selection": Value Change {
        n136 = event-data() -> ("NewVal"=w236:u16)  [unwired: 1 in]
        n137 = case shown="0, Default" w236 {
          tunnel: w235 -> [w238 w240]
          tunnel: [w237 w239] -> w234
          frame 0, Default {
            n138 = Unbundle By Name(w238) -> ("X Scale.FString"=w237:string)
          }
          frame 1 {
            n139 = Unbundle By Name(w240) -> ("Y Scale.FString"=w239:string)
          }
        }
        n140 = call <vilib>:"svx_Orbit From FString.vi"("Format string"=w234) -> ("trailing zeros"=w230:bool, "Precision Type"=w231:u16, "Digits"=w232:u8, "Type"=w233:i32)  [unwired: 7 in]
        n141 = local write "Hide trailing zeros"(w230) -> ()
        n142 = local write "Precision Type"(w231) -> ()
        n143 = local write "Digits"(w232) -> ()
        n144 = local write "Type"(w233) -> ()
      }
      event "Plot.Line Style": Value Change {
        w241 = T14[] [enum."[Plot] Data Point"] items=["None", "[Axis] Range", "[Plot] Image", "[Plot] Tacho Point", "[Plot] Grid and BG", "[Cursor] Cursor Info", "[Legend] Pair Strings", "[Data] Plot Data", "[Legend] Checkbox", "[Layout] Update", "[Legend] Tree Open", "[Layout] Legend Visible", "[Plot] Data Point", "[Axis] Axis and Label", "[Axis] Format String", "[Cursor] Appearance", "[Cursor] Index", "[Legend] Color", "[Layout] Min Pane Size", "[Data] Legend Strings"] ("event")
        w250 = bool[] []
        n145 = event-data() -> ("CtlRef"=w245:refnum<vi>, "OldVal"=w251:T9, "NewVal"=w252:T9)  [unwired: 1 in]
        n146 = Variant To Data(type=w250, Variant=w252) -> (data=w249:bool[])  [unwired: 1 in, 1 out]
        n147 = Variant To Data(type=w250, Variant=w251) -> (data=w248:bool[])  [unwired: 1 in, 1 out]
        n148 = Exclusive Or(1:w249, 2:w248) -> (0:w247:bool[])
        n149 = Search 1D Array(1D array=w247, element=TRUE) -> (index of element=w242:i32)  [unwired: 1 in]
        n150 = Bundle By Name(cluster=w244, "Plot.Line Style"=w242) -> (w243:T4)
        n151 = call <vilib>:"svx_Orbit Manage Cluster.vi"("index"=w242, "Clust Refnum"=w245) -> ()  [unwired: 10 in]
      }
      event "Plot.Line Width": Value Change {
        w253 = T14[] [enum."[Plot] Data Point"] items=["None", "[Axis] Range", "[Plot] Image", "[Plot] Tacho Point", "[Plot] Grid and BG", "[Cursor] Cursor Info", "[Legend] Pair Strings", "[Data] Plot Data", "[Legend] Checkbox", "[Layout] Update", "[Legend] Tree Open", "[Layout] Legend Visible", "[Plot] Data Point", "[Axis] Axis and Label", "[Axis] Format String", "[Cursor] Appearance", "[Cursor] Index", "[Legend] Color", "[Layout] Min Pane Size", "[Data] Legend Strings"] ("event")
        w264 = bool[] []
        n152 = event-data() -> ("CtlRef"=w254:refnum<vi>, "OldVal"=w255:T10, "NewVal"=w256:T10)  [unwired: 1 in]
        n153 = Variant To Data(type=w264, Variant=w256) -> (data=w263:bool[])  [unwired: 1 in, 1 out]
        n154 = Variant To Data(type=w264, Variant=w255) -> (data=w262:bool[])  [unwired: 1 in, 1 out]
        n155 = Exclusive Or(1:w263, 2:w262) -> (0:w261:bool[])
        n156 = Search 1D Array(1D array=w261, element=TRUE) -> (index of element=w257:i32)  [unwired: 1 in]
        n157 = Bundle By Name(cluster=w259, "Plot.Line Width"=w257) -> (w258:T4)
        n158 = call <vilib>:"svx_Orbit Manage Cluster.vi"("index"=w257, "Clust Refnum"=w254) -> ()  [unwired: 10 in]
      }
      event "Plot.Point Style": Value Change {
        w265 = T14[] [enum."[Plot] Data Point"] items=["None", "[Axis] Range", "[Plot] Image", "[Plot] Tacho Point", "[Plot] Grid and BG", "[Cursor] Cursor Info", "[Legend] Pair Strings", "[Data] Plot Data", "[Legend] Checkbox", "[Layout] Update", "[Legend] Tree Open", "[Layout] Legend Visible", "[Plot] Data Point", "[Axis] Axis and Label", "[Axis] Format String", "[Cursor] Appearance", "[Cursor] Index", "[Legend] Color", "[Layout] Min Pane Size", "[Data] Legend Strings"] ("event")
        w276 = bool[] []
        n159 = event-data() -> ("CtlRef"=w266:refnum<vi>, "OldVal"=w267:T8, "NewVal"=w268:T8)  [unwired: 1 in]
        n160 = Variant To Data(type=w276, Variant=w268) -> (data=w275:bool[])  [unwired: 1 in, 1 out]
        n161 = Variant To Data(type=w276, Variant=w267) -> (data=w274:bool[])  [unwired: 1 in, 1 out]
        n162 = Exclusive Or(1:w275, 2:w274) -> (0:w273:bool[])
        n163 = Search 1D Array(1D array=w273, element=TRUE) -> (index of element=w269:i32)  [unwired: 1 in]
        n164 = Bundle By Name(cluster=w271, "Plot.Point Style"=w269) -> (w270:T4)
        n165 = call <vilib>:"svx_Orbit Manage Cluster.vi"("index"=w269, "Clust Refnum"=w266) -> ()  [unwired: 10 in]
      }
      event "Line.Color": Value Change {
        w277 = T14[] [enum."[Plot] Data Point"] items=["None", "[Axis] Range", "[Plot] Image", "[Plot] Tacho Point", "[Plot] Grid and BG", "[Cursor] Cursor Info", "[Legend] Pair Strings", "[Data] Plot Data", "[Legend] Checkbox", "[Layout] Update", "[Legend] Tree Open", "[Layout] Legend Visible", "[Plot] Data Point", "[Axis] Axis and Label", "[Axis] Format String", "[Cursor] Appearance", "[Cursor] Index", "[Legend] Color", "[Layout] Min Pane Size", "[Data] Legend Strings"] ("event")
        n166 = event-data() -> ("NewVal"=w278:u32)  [unwired: 1 in]
        n167 = Bundle By Name(cluster=w280, "Plot.Plot Color"=w278) -> (w279:T4)
      }
      event "Point/Fill.Color": Value Change {
        w281 = T14[] [enum."[Plot] Data Point"] items=["None", "[Axis] Range", "[Plot] Image", "[Plot] Tacho Point", "[Plot] Grid and BG", "[Cursor] Cursor Info", "[Legend] Pair Strings", "[Data] Plot Data", "[Legend] Checkbox", "[Layout] Update", "[Legend] Tree Open", "[Layout] Legend Visible", "[Plot] Data Point", "[Axis] Axis and Label", "[Axis] Format String", "[Cursor] Appearance", "[Cursor] Index", "[Legend] Color", "[Layout] Min Pane Size", "[Data] Legend Strings"] ("event")
        n168 = event-data() -> ("NewVal"=w282:u32)  [unwired: 1 in]
        n169 = Bundle By Name(cluster=w284, "Plot.Point/fill"=w282) -> (w283:T4)
      }
      event "Trigger Point.Color": Value Change {
        w285 = T14[] [enum."[Plot] Tacho Point"] items=["None", "[Axis] Range", "[Plot] Image", "[Plot] Tacho Point", "[Plot] Grid and BG", "[Cursor] Cursor Info", "[Legend] Pair Strings", "[Data] Plot Data", "[Legend] Checkbox", "[Layout] Update", "[Legend] Tree Open", "[Layout] Legend Visible", "[Plot] Data Point", "[Axis] Axis and Label", "[Axis] Format String", "[Cursor] Appearance", "[Cursor] Index", "[Legend] Color", "[Layout] Min Pane Size", "[Data] Legend Strings"] ("event")
        n170 = event-data() -> ("NewVal"=w286:u32)  [unwired: 1 in]
        n171 = Bundle By Name(cluster=w288, "Tacho Point Color"=w286) -> (w287:T4)
      }
      event "Scale Name": Value Change {
        w289 = T14[] [enum."[Axis] Axis and Label"] items=["None", "[Axis] Range", "[Plot] Image", "[Plot] Tacho Point", "[Plot] Grid and BG", "[Cursor] Cursor Info", "[Legend] Pair Strings", "[Data] Plot Data", "[Legend] Checkbox", "[Layout] Update", "[Legend] Tree Open", "[Layout] Legend Visible", "[Plot] Data Point", "[Axis] Axis and Label", "[Axis] Format String", "[Cursor] Appearance", "[Cursor] Index", "[Legend] Color", "[Layout] Min Pane Size", "[Data] Legend Strings"] ("event")
        n172 = event-data() -> ("NewVal"=w292:string)  [unwired: 1 in]
        n173 = local read "Scale Selection"() -> (w293:u16)
        n174 = property on="Scale Selection" class="Ring (strict)"() -> ("Strings []"=w295:string[])  [unwired: 2 in, 2 out]
        n175 = case shown="0, Default" w293 {
          tunnel: w292 -> [w298 w303]
          tunnel: w297 -> [w301 w305]
          tunnel: [w300 w304] -> w296
          tunnel: [" (X-Axis)" ("string") " (Y-Axis)" ("string")] -> w290
          frame 0, Default {
            n176 = Bundle By Name(cluster=w301, "X Scale.Name"=w298) -> (w300:T4)
          }
          frame 1 {
            n177 = Bundle By Name(cluster=w305, "Y Scale.Name"=w303) -> (w304:T4)
          }
        }
        n178 = Concatenate Strings(w292, w290) -> (w294:string)
        n179 = Replace Array Subset(array=w295, new element=w294, index=w293) -> (w291:string[])
        n180 = property on="Scale Selection" class="Ring (strict)"("Strings []"=w291) -> ()  [unwired: 2 in, 2 out]
        n181 = property on="Format Selection" class="Ring (strict)"("Strings []"=w291) -> ()  [unwired: 2 in, 2 out]
      }
      event "Scale Label.Visible": Value Change {
        w306 = T14[] [enum."[Axis] Axis and Label"] items=["None", "[Axis] Range", "[Plot] Image", "[Plot] Tacho Point", "[Plot] Grid and BG", "[Cursor] Cursor Info", "[Legend] Pair Strings", "[Data] Plot Data", "[Legend] Checkbox", "[Layout] Update", "[Legend] Tree Open", "[Layout] Legend Visible", "[Plot] Data Point", "[Axis] Axis and Label", "[Axis] Format String", "[Cursor] Appearance", "[Cursor] Index", "[Legend] Color", "[Layout] Min Pane Size", "[Data] Legend Strings"] ("event")
        n182 = event-data() -> ("NewVal"=w308:bool)  [unwired: 1 in]
        n183 = local read "Scale Selection"() -> (w307:u16)
        n184 = case shown="1" w307 {
          tunnel: w308 -> [w311 w314]
          tunnel: w310 -> [w313 w316]
          tunnel: [w312 w315] -> w309
          frame 0, Default {
            n185 = Bundle By Name(cluster=w313, "X Scale.Label Visible"=w311) -> (w312:T4)
          }
          frame 1 {
            n186 = Bundle By Name(cluster=w316, "Y Scale.Label Visible"=w314) -> (w315:T4)
          }
        }
      }
      event "Scale.Visible": Value Change {
        w317 = T14[] [enum."[Axis] Axis and Label"] items=["None", "[Axis] Range", "[Plot] Image", "[Plot] Tacho Point", "[Plot] Grid and BG", "[Cursor] Cursor Info", "[Legend] Pair Strings", "[Data] Plot Data", "[Legend] Checkbox", "[Layout] Update", "[Legend] Tree Open", "[Layout] Legend Visible", "[Plot] Data Point", "[Axis] Axis and Label", "[Axis] Format String", "[Cursor] Appearance", "[Cursor] Index", "[Legend] Color", "[Layout] Min Pane Size", "[Data] Legend Strings"] ("event")
        n187 = event-data() -> ("NewVal"=w319:bool)  [unwired: 1 in]
        n188 = local read "Scale Selection"() -> (w318:u16)
        n189 = case shown="0, Default" w318 {
          tunnel: w319 -> [w322 w325]
          tunnel: w321 -> [w324 w327]
          tunnel: [w323 w326] -> w320
          frame 0, Default {
            n190 = Bundle By Name(cluster=w324, "X Scale.Scale Visible"=w322) -> (w323:T4)
          }
          frame 1 {
            n191 = Bundle By Name(cluster=w327, "Y Scale.Scale Visible"=w325) -> (w326:T4)
          }
        }
      }
      event "Scale Fit": Value Change {
        n192 = event-data() -> ("NewVal"=w330:bool)  [unwired: 1 in]
        n193 = Boolean To (0,1)(Boolean=w330) -> (0, 1=w336:i16)
        n194 = Bundle By Name(cluster=w331, "Autoscale"=w330) -> (w332:T4)
        n195 = Add(x=w336, y=w336) -> (x+y=w334:i16)
        n196 = property on="Minimum" class="DigNum (strict)"("Disabled"=w334) -> ()  [unwired: 2 in, 2 out]
        n197 = property on="Maximum" class="DigNum (strict)"("Disabled"=w334) -> ()  [unwired: 2 in, 2 out]
        n198 = call <vilib>:"svx_Orbit Autoscale.vi"("Display State In"=w332, 7:"Orbit Plot"=w333, 11:"Orbit Plot"=w337) -> ("Display State Out"=w329:T4)  [unwired: 8 in]
        n199 = Unbundle By Name(w329) -> ("Axis Maximum"=w328:dbl)
        n200 = Negate(x=w328) -> (-x=w335:dbl)
        n201 = local write "Minimum"(w335) -> ()
        n202 = local write "Maximum"(w328) -> ()
      }
      event "Minimum", "Maximum": Value Change {
        w338 = T14[] [enum."[Axis] Range"] items=["None", "[Axis] Range", "[Plot] Image", "[Plot] Tacho Point", "[Plot] Grid and BG", "[Cursor] Cursor Info", "[Legend] Pair Strings", "[Data] Plot Data", "[Legend] Checkbox", "[Layout] Update", "[Legend] Tree Open", "[Layout] Legend Visible", "[Plot] Data Point", "[Axis] Axis and Label", "[Axis] Format String", "[Cursor] Appearance", "[Cursor] Index", "[Legend] Color", "[Layout] Min Pane Size", "[Data] Legend Strings"] ("event")
        n203 = event-data() -> ("NewVal"=w344:dbl)  [unwired: 1 in]
        n204 = Absolute Value(x=w344) -> (abs(x)=w341:dbl)
        n205 = Negate(x=w341) -> (-x=w342:dbl)
        n206 = local write "Minimum"(w342) -> ()
        n207 = local write "Maximum"(w341) -> ()
        n208 = Bundle By Name(cluster=w343, "Axis Maximum"=w341, "Autoscale"=FALSE) -> (w340:T4)
      }
      event "XGrid Style": Value Change {
        w348 = T14[] [enum."[Plot] Grid and BG"] items=["None", "[Axis] Range", "[Plot] Image", "[Plot] Tacho Point", "[Plot] Grid and BG", "[Cursor] Cursor Info", "[Legend] Pair Strings", "[Data] Plot Data", "[Legend] Checkbox", "[Layout] Update", "[Legend] Tree Open", "[Layout] Legend Visible", "[Plot] Data Point", "[Axis] Axis and Label", "[Axis] Format String", "[Cursor] Appearance", "[Cursor] Index", "[Legend] Color", "[Layout] Min Pane Size", "[Data] Legend Strings"] ("event")
        n209 = event-data() -> ("NewVal"=w345:u16)  [unwired: 1 in]
        n210 = case shown="1" w345 {
          tunnel: [w351 u8 0 ("Disabled") w354] -> w347
          tunnel: [w351 u8 2 ("Disabled") w354] -> w346
          frame 0, Default {
            w351 = u8 2 ("Disabled")
          }
          frame 1 {
          }
          frame 2 {
            w354 = u8 0 ("Disabled")
          }
        }
        n211 = property on="Major Grid.Color" class="ColBox"("Disabled"=w347) -> ()  [unwired: 2 in, 2 out]
        n212 = property on="Minor Grid.Color" class="ColBox"("Disabled"=w346) -> ()  [unwired: 2 in, 2 out]
        n213 = Bundle By Name(cluster=w349, "X Scale.Grid Style"=w345) -> (w350:T4)
      }
      event "YGrid Style": Value Change {
        w355 = T14[] [enum."[Plot] Grid and BG"] items=["None", "[Axis] Range", "[Plot] Image", "[Plot] Tacho Point", "[Plot] Grid and BG", "[Cursor] Cursor Info", "[Legend] Pair Strings", "[Data] Plot Data", "[Legend] Checkbox", "[Layout] Update", "[Legend] Tree Open", "[Layout] Legend Visible", "[Plot] Data Point", "[Axis] Axis and Label", "[Axis] Format String", "[Cursor] Appearance", "[Cursor] Index", "[Legend] Color", "[Layout] Min Pane Size", "[Data] Legend Strings"] ("event")
        n214 = event-data() -> ("NewVal"=w356:u16)  [unwired: 1 in]
        n215 = case shown="2" w356 {
          tunnel: [w361 u8 0 ("Disabled") w364] -> w358
          tunnel: [w361 u8 2 ("Disabled") w364] -> w357
          frame 0, Default {
            w361 = u8 2 ("Disabled")
          }
          frame 1 {
          }
          frame 2 {
            w364 = u8 0 ("Disabled")
          }
        }
        n216 = property on="Major Grid.Color" class="ColBox"("Disabled"=w358) -> ()  [unwired: 2 in, 2 out]
        n217 = property on="Minor Grid.Color" class="ColBox"("Disabled"=w357) -> ()  [unwired: 2 in, 2 out]
        n218 = Bundle By Name(cluster=w359, "Y Scale.Grid Style"=w356) -> (w360:T4)
      }
      event "Major Grid.Color": Value Change {
        w365 = T14[] [enum."[Plot] Grid and BG"] items=["None", "[Axis] Range", "[Plot] Image", "[Plot] Tacho Point", "[Plot] Grid and BG", "[Cursor] Cursor Info", "[Legend] Pair Strings", "[Data] Plot Data", "[Legend] Checkbox", "[Layout] Update", "[Legend] Tree Open", "[Layout] Legend Visible", "[Plot] Data Point", "[Axis] Axis and Label", "[Axis] Format String", "[Cursor] Appearance", "[Cursor] Index", "[Legend] Color", "[Layout] Min Pane Size", "[Data] Legend Strings"] ("event")
        n219 = event-data() -> ("NewVal"=w367:u32)  [unwired: 1 in]
        n220 = local read "Scale Selection"() -> (w366:u16)
        n221 = case shown="0, Default" w366 {
          tunnel: w369 -> [w372 w375]
          tunnel: [w371 w374] -> w368
          tunnel: w367 -> [w370 w373]
          frame 0, Default {
            n222 = Bundle By Name(cluster=w372, "X Scale.Major Color"=w370) -> (w371:T4)
          }
          frame 1 {
            n223 = Bundle By Name(cluster=w375, "Y Scale.Major Color"=w373) -> (w374:T4)
          }
        }
      }
      event "Minor Grid.Color": Value Change {
        w376 = T14[] [enum."[Plot] Grid and BG"] items=["None", "[Axis] Range", "[Plot] Image", "[Plot] Tacho Point", "[Plot] Grid and BG", "[Cursor] Cursor Info", "[Legend] Pair Strings", "[Data] Plot Data", "[Legend] Checkbox", "[Layout] Update", "[Legend] Tree Open", "[Layout] Legend Visible", "[Plot] Data Point", "[Axis] Axis and Label", "[Axis] Format String", "[Cursor] Appearance", "[Cursor] Index", "[Legend] Color", "[Layout] Min Pane Size", "[Data] Legend Strings"] ("event")
        n224 = event-data() -> ("NewVal"=w378:u32)  [unwired: 1 in]
        n225 = local read "Scale Selection"() -> (w377:u16)
        n226 = case shown="1" w377 {
          tunnel: w380 -> [w383 w386]
          tunnel: [w382 w385] -> w379
          tunnel: w378 -> [w381 w384]
          frame 0, Default {
            n227 = Bundle By Name(cluster=w383, "X Scale.Minor Color"=w381) -> (w382:T4)
          }
          frame 1 {
            n228 = Bundle By Name(cluster=w386, "Y Scale.Minor Color"=w384) -> (w385:T4)
          }
        }
      }
      event "Scale Selection": Value Change {
        n229 = event-data() -> ("NewVal"=w390:u16)  [unwired: 1 in]
        n230 = case shown="1" w390 {
          tunnel: [w413 w424] -> w387
          tunnel: [w412 w423] -> w397
          tunnel: [w411 w422] -> w395
          tunnel: [w410 w421] -> w394
          tunnel: [w409 w420] -> w393
          tunnel: [w408 w419] -> w392
          tunnel: [w407 w418] -> w391
          tunnel: w389 -> [w406 w417]
          tunnel: [w403 w414] -> w388
          frame 0, Default {
            n231 = Unbundle By Name(w406) -> ("X Scale.Name"=w407:string, "X Scale.Label Visible"=w408:bool, "X Scale.Scale Visible"=w409:bool, "X Scale.Major Color"=w410:u32, "X Scale.Minor Color"=w411:u32, "Autoscale"=w413:bool, "Axis Maximum"=w412:dbl, "X Scale.Grid Style"=w403:u16)
            n232 = property on="XGrid Style" class="Ring (strict)"("Visible"=TRUE) -> ()  [unwired: 2 in, 2 out]
            n233 = local write "XGrid Style"(w403) -> ()
            n234 = property on="YGrid Style" class="Ring (strict)"("Visible"=FALSE) -> ()  [unwired: 2 in, 2 out]
          }
          frame 1 {
            n235 = Unbundle By Name(w417) -> ("Y Scale.Name"=w418:string, "Y Scale.Label Visible"=w419:bool, "Y Scale.Scale Visible"=w420:bool, "Y Scale.Major Color"=w421:u32, "Y Scale.Minor Color"=w422:u32, "Autoscale"=w424:bool, "Axis Maximum"=w423:dbl, "Y Scale.Grid Style"=w414:u16)
            n236 = property on="XGrid Style" class="Ring (strict)"("Visible"=FALSE) -> ()  [unwired: 2 in, 2 out]
            n237 = local write "YGrid Style"(w414) -> ()
            n238 = property on="YGrid Style" class="Ring (strict)"("Visible"=TRUE) -> ()  [unwired: 2 in, 2 out]
          }
        }
        n239 = Negate(x=w397) -> (-x=w396:dbl)
        n240 = local write "Minimum"(w396) -> ()
        n241 = local write "Maximum"(w397) -> ()
        n242 = local write "Scale Name"(w391) -> ()
        n243 = local write "Scale.Visible"(w393) -> ()
        n244 = local write "Minor Grid.Color"(w395) -> ()
        n245 = case shown="2" w388 {
          tunnel: [w425 u8 0 ("Disabled") w428] -> w401
          tunnel: [w425 u8 2 ("Disabled") w428] -> w402
          frame 0, Default {
            w425 = u8 2 ("Disabled")
          }
          frame 1 {
          }
          frame 2 {
            w428 = u8 0 ("Disabled")
          }
        }
        n246 = Select(t=u8 2 ("Disabled"), s=w387, f=u8 0) -> (s? t:f=w400:u8)
        n247 = local write "Scale Label.Visible"(w392) -> ()
        n248 = local write "Major Grid.Color"(w394) -> ()
        n249 = local write "Scale Fit"(w387) -> ()
        n250 = property on="Minimum" class="DigNum (strict)"("Disabled"=w400) -> ()  [unwired: 2 in, 2 out]
        n251 = property on="Maximum" class="DigNum (strict)"("Disabled"=w400) -> ()  [unwired: 2 in, 2 out]
        n252 = property on="Major Grid.Color" class="ColBox"("Disabled"=w401) -> ()  [unwired: 2 in, 2 out]
        n253 = property on="Minor Grid.Color" class="ColBox"("Disabled"=w402) -> ()  [unwired: 2 in, 2 out]
      }
      event "Cursor.Line Style": Value Change {
        w429 = T14[] [enum."[Cursor] Appearance"] items=["None", "[Axis] Range", "[Plot] Image", "[Plot] Tacho Point", "[Plot] Grid and BG", "[Cursor] Cursor Info", "[Legend] Pair Strings", "[Data] Plot Data", "[Legend] Checkbox", "[Layout] Update", "[Legend] Tree Open", "[Layout] Legend Visible", "[Plot] Data Point", "[Axis] Axis and Label", "[Axis] Format String", "[Cursor] Appearance", "[Cursor] Index", "[Legend] Color", "[Layout] Min Pane Size", "[Data] Legend Strings"] ("event")
        w440 = bool[] []
        n254 = event-data() -> ("CtlRef"=w430:refnum<vi>, "OldVal"=w431:T9, "NewVal"=w432:T9)  [unwired: 1 in]
        n255 = Variant To Data(type=w440, Variant=w432) -> (data=w439:bool[])  [unwired: 1 in, 1 out]
        n256 = Variant To Data(type=w440, Variant=w431) -> (data=w438:bool[])  [unwired: 1 in, 1 out]
        n257 = Exclusive Or(1:w439, 2:w438) -> (0:w437:bool[])
        n258 = Search 1D Array(1D array=w437, element=TRUE) -> (index of element=w433:i32)  [unwired: 1 in]
        n259 = Bundle By Name(cluster=w435, "Cursor.Cursor Line Style"=w433) -> (w434:T4)
        n260 = call <vilib>:"svx_Orbit Manage Cluster.vi"("index"=w433, "Clust Refnum"=w430) -> ()  [unwired: 10 in]
      }
      event "Cursor.Line Width": Value Change {
        w441 = T14[] [enum."[Cursor] Appearance"] items=["None", "[Axis] Range", "[Plot] Image", "[Plot] Tacho Point", "[Plot] Grid and BG", "[Cursor] Cursor Info", "[Legend] Pair Strings", "[Data] Plot Data", "[Legend] Checkbox", "[Layout] Update", "[Legend] Tree Open", "[Layout] Legend Visible", "[Plot] Data Point", "[Axis] Axis and Label", "[Axis] Format String", "[Cursor] Appearance", "[Cursor] Index", "[Legend] Color", "[Layout] Min Pane Size", "[Data] Legend Strings"] ("event")
        w452 = bool[] []
        n261 = event-data() -> ("CtlRef"=w442:refnum<vi>, "OldVal"=w443:T10, "NewVal"=w444:T10)  [unwired: 1 in]
        n262 = Variant To Data(type=w452, Variant=w444) -> (data=w451:bool[])  [unwired: 1 in, 1 out]
        n263 = Variant To Data(type=w452, Variant=w443) -> (data=w450:bool[])  [unwired: 1 in, 1 out]
        n264 = Exclusive Or(1:w451, 2:w450) -> (0:w449:bool[])
        n265 = Search 1D Array(1D array=w449, element=TRUE) -> (index of element=w445:i32)  [unwired: 1 in]
        n266 = Bundle By Name(cluster=w447, "Cursor.Cursor Line Width"=w445) -> (w446:T4)
        n267 = call <vilib>:"svx_Orbit Manage Cluster.vi"("index"=w445, "Clust Refnum"=w442) -> ()  [unwired: 10 in]
      }
      event "Cursor.Point Style": Value Change {
        w453 = T14[] [enum."[Cursor] Appearance"] items=["None", "[Axis] Range", "[Plot] Image", "[Plot] Tacho Point", "[Plot] Grid and BG", "[Cursor] Cursor Info", "[Legend] Pair Strings", "[Data] Plot Data", "[Legend] Checkbox", "[Layout] Update", "[Legend] Tree Open", "[Layout] Legend Visible", "[Plot] Data Point", "[Axis] Axis and Label", "[Axis] Format String", "[Cursor] Appearance", "[Cursor] Index", "[Legend] Color", "[Layout] Min Pane Size", "[Data] Legend Strings"] ("event")
        w464 = bool[] []
        n268 = event-data() -> ("CtlRef"=w454:refnum<vi>, "OldVal"=w455:T8, "NewVal"=w456:T8)  [unwired: 1 in]
        n269 = Variant To Data(type=w464, Variant=w456) -> (data=w463:bool[])  [unwired: 1 in, 1 out]
        n270 = Variant To Data(type=w464, Variant=w455) -> (data=w462:bool[])  [unwired: 1 in, 1 out]
        n271 = Exclusive Or(1:w463, 2:w462) -> (0:w461:bool[])
        n272 = Search 1D Array(1D array=w461, element=TRUE) -> (index of element=w457:i32)  [unwired: 1 in]
        n273 = Bundle By Name(cluster=w459, "Cursor.Cursor Point Style"=w457) -> (w458:T4)
        n274 = call <vilib>:"svx_Orbit Manage Cluster.vi"("index"=w457, "Clust Refnum"=w454) -> ()  [unwired: 10 in]
      }
      event "Cursor.Style": Value Change {
        w465 = T14[] [enum."[Cursor] Appearance"] items=["None", "[Axis] Range", "[Plot] Image", "[Plot] Tacho Point", "[Plot] Grid and BG", "[Cursor] Cursor Info", "[Legend] Pair Strings", "[Data] Plot Data", "[Legend] Checkbox", "[Layout] Update", "[Legend] Tree Open", "[Layout] Legend Visible", "[Plot] Data Point", "[Axis] Axis and Label", "[Axis] Format String", "[Cursor] Appearance", "[Cursor] Index", "[Legend] Color", "[Layout] Min Pane Size", "[Data] Legend Strings"] ("event")
        w476 = bool[] []
        n275 = event-data() -> ("CtlRef"=w466:refnum<vi>, "OldVal"=w467:T11, "NewVal"=w468:T11)  [unwired: 1 in]
        n276 = Variant To Data(type=w476, Variant=w468) -> (data=w475:bool[])  [unwired: 1 in, 1 out]
        n277 = Variant To Data(type=w476, Variant=w467) -> (data=w474:bool[])  [unwired: 1 in, 1 out]
        n278 = Exclusive Or(1:w475, 2:w474) -> (0:w473:bool[])
        n279 = Search 1D Array(1D array=w473, element=TRUE) -> (index of element=w469:i32)  [unwired: 1 in]
        n280 = Bundle By Name(cluster=w471, "Cursor.Cursor Style"=w469) -> (w470:T4)
        n281 = call <vilib>:"svx_Orbit Manage Cluster.vi"("index"=w469, "Clust Refnum"=w466) -> ()  [unwired: 10 in]
      }
      event "Cursor Info.Visible": Value Change {
        w477 = T14[] [enum."[Cursor] Cursor Info"] items=["None", "[Axis] Range", "[Plot] Image", "[Plot] Tacho Point", "[Plot] Grid and BG", "[Cursor] Cursor Info", "[Legend] Pair Strings", "[Data] Plot Data", "[Legend] Checkbox", "[Layout] Update", "[Legend] Tree Open", "[Layout] Legend Visible", "[Plot] Data Point", "[Axis] Axis and Label", "[Axis] Format String", "[Cursor] Appearance", "[Cursor] Index", "[Legend] Color", "[Layout] Min Pane Size", "[Data] Legend Strings"] ("event")
        n282 = event-data() -> ("NewVal"=w479:bool)  [unwired: 1 in]
        n283 = Select(t=u8 0 ("Disabled"), s=w479, f=u8 2) -> (s? t:f=w478:u8)
        n284 = Bundle By Name(cluster=w483, "Cursor.Cursor Name Visible"=w479) -> (w482:T4)
        n285 = property on="Cursor Info Position.Lock" class="Bool (strict)"("Disabled"=w478) -> ()  [unwired: 2 in, 2 out]
      }
      event "Cursor.Visible": Value Change {
        w486 = T14[] [enum."[Cursor] Cursor Info"] items=["None", "[Axis] Range", "[Plot] Image", "[Plot] Tacho Point", "[Plot] Grid and BG", "[Cursor] Cursor Info", "[Legend] Pair Strings", "[Data] Plot Data", "[Legend] Checkbox", "[Layout] Update", "[Legend] Tree Open", "[Layout] Legend Visible", "[Plot] Data Point", "[Axis] Axis and Label", "[Axis] Format String", "[Cursor] Appearance", "[Cursor] Index", "[Legend] Color", "[Layout] Min Pane Size", "[Data] Legend Strings"] ("event")
        n286 = event-data() -> ("NewVal"=w491:bool)  [unwired: 1 in]
        n287 = Unbundle By Name(w485) -> ("Cursor.Cursor Name Visible"=w484:bool)
        n288 = And(x=w491, y=w484) -> (x .and. y?=w487:bool)
        n289 = Select(t=u8 0 ("Disabled"), s=w491, f=u8 2) -> (s? t:f=w492:u8)
        n290 = Select(t=u8 0 ("Disabled"), s=w487, f=u8 2) -> (s? t:f=w488:u8)
        n291 = Bundle By Name(cluster=w485, "Cursor.Cursor Visible"=w491) -> (w495:T4)
        n292 = property on="Cursor Info.Visible" class="Bool (strict)"("Disabled"=w492) -> ()  [unwired: 2 in, 2 out]
        n293 = property on="Cursor Info Position.Lock" class="Bool (strict)"("Disabled"=w488) -> ()  [unwired: 2 in, 2 out]
      }
      event "Cursor.Color": Value Change {
        w496 = T14[] [enum."[Cursor] Appearance", enum."[Cursor] Cursor Info"] items=["None", "[Axis] Range", "[Plot] Image", "[Plot] Tacho Point", "[Plot] Grid and BG", "[Cursor] Cursor Info", "[Legend] Pair Strings", "[Data] Plot Data", "[Legend] Checkbox", "[Layout] Update", "[Legend] Tree Open", "[Layout] Legend Visible", "[Plot] Data Point", "[Axis] Axis and Label", "[Axis] Format String", "[Cursor] Appearance", "[Cursor] Index", "[Legend] Color", "[Layout] Min Pane Size", "[Data] Legend Strings"] ("event")
        n294 = event-data() -> ("NewVal"=w497:u32)  [unwired: 1 in]
        n295 = Bundle By Name(cluster=w499, "Cursor.Cursor Color"=w497) -> (w498:T4)
      }
      event "Cursor Info Position.Lock": Value Change {
        w500 = T14[] [enum."[Cursor] Cursor Info"] items=["None", "[Axis] Range", "[Plot] Image", "[Plot] Tacho Point", "[Plot] Grid and BG", "[Cursor] Cursor Info", "[Legend] Pair Strings", "[Data] Plot Data", "[Legend] Checkbox", "[Layout] Update", "[Legend] Tree Open", "[Layout] Legend Visible", "[Plot] Data Point", "[Axis] Axis and Label", "[Axis] Format String", "[Cursor] Appearance", "[Cursor] Index", "[Legend] Color", "[Layout] Min Pane Size", "[Data] Legend Strings"] ("event")
        n296 = event-data() -> ("NewVal"=w502:bool)  [unwired: 1 in]
        n297 = Bundle By Name(cluster=w503, "Cursor.Cursor Lock"=w502) -> (w501:T4)
      }
      event "Description": Value Change {
        n298 = event-data() -> ("NewVal"=w505:string)  [unwired: 1 in]
        n299 = property class="Ctl"(reference=w506, "Desc"=w505) -> ()  [unwired: 1 in, 2 out]
      }
      event "Tip strip": Value Change {
        n300 = event-data() -> ("NewVal"=w508:string)  [unwired: 1 in]
        n301 = property class="Ctl"(reference=w509, "TipStrip"=w508) -> ()  [unwired: 1 in, 2 out]
      }
    }
    n302 = Unbundle By Name(w125) -> ("Refnum"=w124:refnum<vi>, "Orbit Plot"=w123:refnum<vi>, "Tree"=w122:refnum<vi>, "Cursor Info"=w121:refnum<vi>, "This VI"=w120:refnum<vi>)
    n303 = call <vilib>:"svx_Orbit Exec Commands.vi"("Display State In"=w130, "Data In"=w128, "Commands"=w131, "Container"=w124, "Facade VI"=w120, "Cursor Info"=w121, "Tree"=w122, "Orbit Plot"=w123) -> ("Display State Out"=w129:T4)  [unwired: 3 in]
  }
  "State out" <- w12
  "Action out" <- w4
